vi "oax_Configuration.vi"(8 "error in (no error)":errorcluster) -> (0 "error out":errorcluster, 2 "Bandwidth":T1={"bandwidth"=1.0, "unit"=enum."Order"}, 3 "Windows info":cluster{"window type":u32, "window length":i32}={"window type"=62, "window length"=2048} {"window length" min=2; "window type" items=["None"=0, "Hanning"=1, "Hamming"=2, "Blackman-Harris"=3, "Exact Blackman"=4, "Blackman"=5, "Flat Top"=6, "4 Term B-Harris"=7, "7 Term B-Harris"=8, "Low Sidelobe"=9, "Gaussian"=62]}, 5 "OK?":bool)   [LabVIEW 2017]
panel:
  in  "Cancel":bool
  in  "OK":bool
  in  "Windows Info":cluster{"Window Type":u32, "Window Length":i32}={"Window Type"=62, "Window Length"=2048} {"Window Length" min=2; "Window Type" items=["None"=0, "Hanning"=1, "Hamming"=2, "Blackman-Harris"=3, "Exact Blackman"=4, "Blackman"=5, "Flat Top"=6, "4 Term B-Harris"=7, "7 Term B-Harris"=8, "Low Sidelobe"=9, "Gaussian"=62]}
  in  "Bandwidth":T2={"Bandwidth"=1.0, "Unit"=enum."Order"} {"Bandwidth" min=0.0}
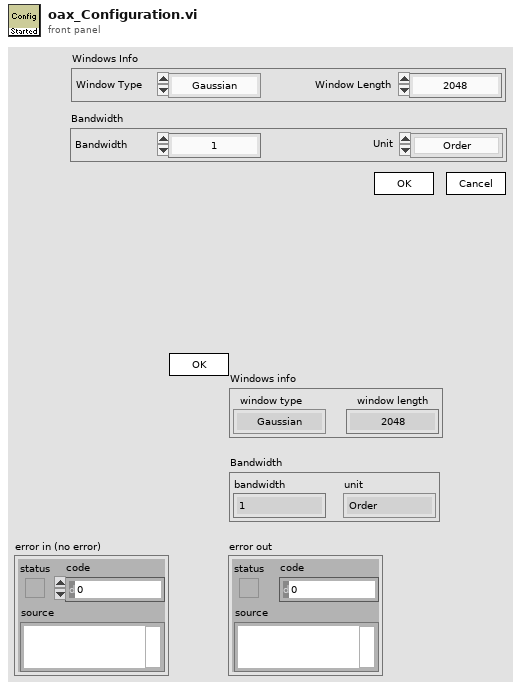
[diagram p1: front panel]
types:
  T1 = cluster{"bandwidth":dbl, "unit":enum16{"Order", "Hz"}}
  T2 = cluster{"Bandwidth":dbl, "Unit":enum16{"Order", "Hz"}}
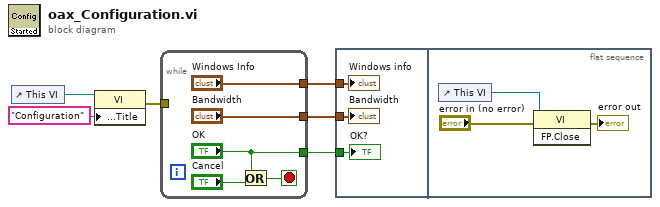
[diagram p0: block diagram]
diagram:
  n1 = control-ref of="This VI"() -> (w3:refnum<vi>)
  n2 = property class="VI"(reference=w3, "Front Panel.Title"="Configuration" ("Front Panel Window:Title")) -> (error out=w1:errorcluster)  [unwired: 1 in, 1 out]
  n3 = while {
    tunnel: ["Windows Info"] -> w6
    tunnel: ["Bandwidth"] -> w5
    tunnel: ["OK"] -> w4
    tunnel: w1 -> [_]
    stop <- w10 stop-if-true
    n4 = Or(x="OK", y="Cancel") -> (x .or. y?=w10:bool)
  }
  n5 = flat-sequence {
    tunnel: w6 -> [w14]
    tunnel: w5 -> [w13]
    tunnel: w4 -> [w12]
    frame #0 {
      "Windows info" <- w14
      "Bandwidth" <- w13
      "OK?" <- w12
    }
    frame #1 {
      n6 = control-ref of="This VI"() -> (w17:refnum<vi>)
      n7 = invoke class="VI" method="FP.Close"(reference=w17, error in="error in (no error)") -> (error out=→"error out":errorcluster)  [unwired: 1 in, 2 out]
    }
  }
